vi "Insert Constant VIs.vi"(7 "Application in":refnum<vi>, 8 "Tree Map in":T1, 9 "Root path":string, 10 "DQMH Lib In":refnum<vi>) -> (0 "Tree Map Out":T1)   [LabVIEW 2019, in "Panther Dashboard.lvlib"]
uses:
  Panther Dashboard.lvlib
  <vilib>/National Instruments/Tree Map/Tree Map.lvlib
  Class/Library/Library.lvclass
  Class/VI/VI.lvclass
  Map Attribute--enum.ctl
  <vilib>/National Instruments/Tree Map/Tree Map Data.ctl
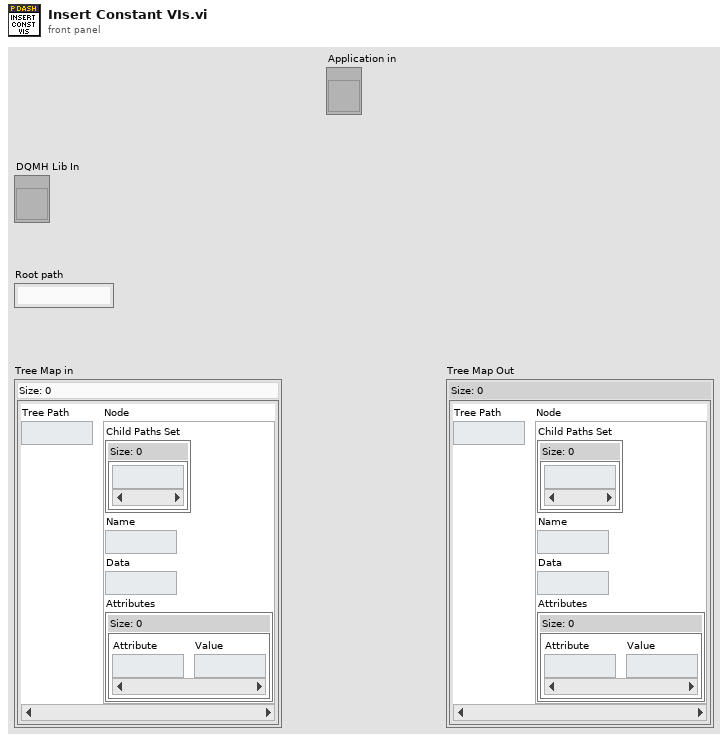
[diagram p1: front panel]
types:
  T1 = typedef "Tree Map.lvlib/Tree Map Data.ctl" = map{string, cluster{"Child Paths Set":set{string}, "Name":string, "Data":string, "Attributes":map{string, string}}}
  T2 = typedef "Panther Dashboard.lvlib/Map Attribute--enum.ctl" = enum16{"Path", "ModuleType", "Module Description", "Dependency?", "Target"}
  T3 = cluster{"status":string, "code":string, "source":string}
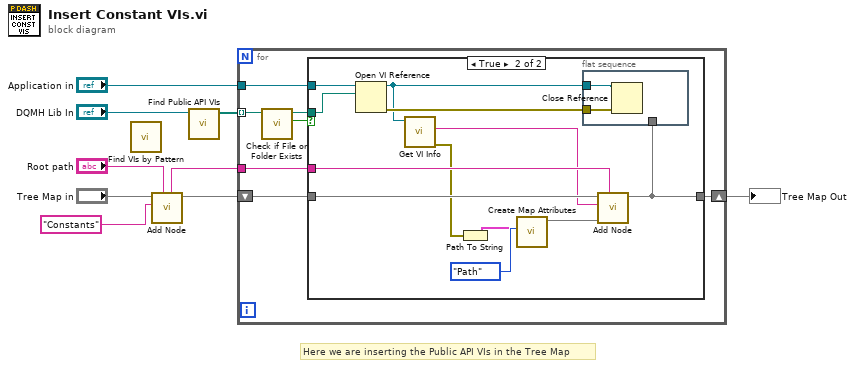
[diagram p0: block diagram]
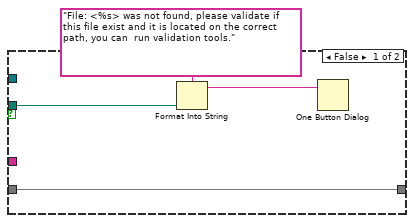
[diagram p2: hidden frame]
diagram:
  # "Here we are inserting the Public API VIs in the Tree Map"
  n1 = call "Find VIs by Pattern.vi"() -> ()  [unwired: 9 in, 3 out]
  n2 = call <vilib>:"Add Node.vi"("Parent Path"="Root path", "New Node Name"="Constants", "Tree Map In"="Tree Map in") -> ("Tree Map Out"=w3:T1, "New Node Path"=w1:string)  [unwired: 6 in, 1 out]
  n3 = call "Find Public API VIs.vi"("Library in"="DQMH Lib In") -> ("Public API VIs Paths"=w8:path[])  [unwired: 9 in, 1 out]
  n4 = for {
    tunnel: "Application in" -> [w16]
    tunnel: w8 -> [w12] mode=indexing
    shift-right: [w15] -> w7
    shift-left: w3 -> [w14]
    tunnel: w1 -> [w13]
    n5 = call <vilib>:"Check if File or Folder Exists.vi"("path"=w12) -> ("file or folder exists?"=w11:bool, "dup path"=w10:path)  [unwired: 8 in, 1 out]
    n6 = case shown="True" w11 {
      tunnel: w16 -> [_ w32]
      tunnel: [w20 w21] -> w15
      tunnel: w14 -> [w20 w31]
      tunnel: w13 -> [_ w30]
      tunnel: w10 -> [w19 w28]
      frame False {
        n7 = Format Into String(format string="File: <%s> was not found, please validate if this file exist and it is located on the correct path, you can  run validation tools.", w19) -> (resulting string=w18:string)  [unwired: 2 in, 1 out]
        n8 = One Button Dialog(message=w18) -> ()  [unwired: 1 in, 1 out]
      }
      frame True {
        n9 = Open VI Reference(application reference (local)=w32, vi path=w28) -> (vi reference=w22:refnum<vi>, error out=w23:errorcluster)  [unwired: 4 in]
        n10 = call "Get VI Info.vi"("VI in"=w22) -> ("error out"=w24:errorcluster, "Plain Name"=w29:string)  [unwired: 6 in, 3 out]
        n11 = Path To String(path=w24) -> (string=w26:T3)
        n12 = call "Create Map Attributes.vi"("Attribute"=w26, "Map Attribute"=Map_Attribute--enum."Path") -> ("Root Attributes"=w25:map{string, string})  [unwired: 9 in]
        n13 = flat-sequence {
          tunnel: w23 -> [w34]
          tunnel: w22 -> [w33]
          tunnel: w21 -> [_]
          frame #0 {
            n14 = Close Reference(reference=w33, error in (no error)=w34) -> ()  [unwired: 1 out]
          }
        }
        n15 = call <vilib>:"Add Node.vi"("Parent Path"=w30, "Attributes"=w25, "New Node Name"=w29, "Tree Map In"=w31) -> ("Tree Map Out"=w21:T1)  [unwired: 5 in, 2 out]
      }
    }
  }
  "Tree Map Out" <- w7
